vi "OL_WaveSaver_rt.vi"() -> ()   [LabVIEW 2020]
uses:
  <vilib>/FPGAPlugInAG/cRIO-9049/niLvFpga_Open_cRIO-9049.vi
  <vilib>/Utility/error.llb/Error Cluster From Error Code.vi
  <vilib>/rvi/errors/niLvFpgaAdjustHostInterfaceError.vi
  <vilib>/FPGAPlugInAG/cRIO-9049/niLvFpga_Run_cRIO-9049.vi
  <vilib>/FPGAPlugInAG/cRIO-9049/niLvFpga_Close_cRIO-9049.vi
  <vilib>/rvi/interface/nirviOpenFPGA/nirviOpenFPGA.xnode
  FPGA Bitfiles/olwavesaverprj_FPGATarget_OLWaveSaverfpga_hKcI+c2eDyU.lvbitx
  OL_WaveSaver_fpga.vi
  <vilib>/rvi/interface/nirviReadWriteControl/nirviReadWriteControl.xnode
  <vilib>/rvi/interface/nirviMethod/nirviMethod.xnode
  <vilib>/rvi/interface/nirviCloseFPGA/nirviCloseFPGA.xnode
  NiFpgaLv.dll
  <vilib>/FPGAPlugInAG/cRIO-9049/niLvFpga_ReadFifo_cRIO-9049.vi
  <vilib>/rvi/errors/niLvFpgaMergeErrorWithErrorCode.vi
panel:
  in  "Filename":path=path "/home/lvuser/natinst/LABVIEWData/OL_PSD_Map_180.lvm"
  out "0":sgl[](graph)
  out "Sum":sgl[](graph)
  out "Time string":string="11/17/2021 15:18:20.858831"
  out "Filename Out":path=path "/home/lvuser/natinst/LABVIEWData/OL_PSD_Dark_5kHz.lvm"
  in  "decimation":i16=25
  in  "Enable":bool
  out "Saving Data":bool
  out "DeltaX":sgl[](graph)
  out "Elements Remaining":u32
  out "DeltaY":sgl[](graph)
  in  "Number of Elements":u32=400
  in  "stop":bool
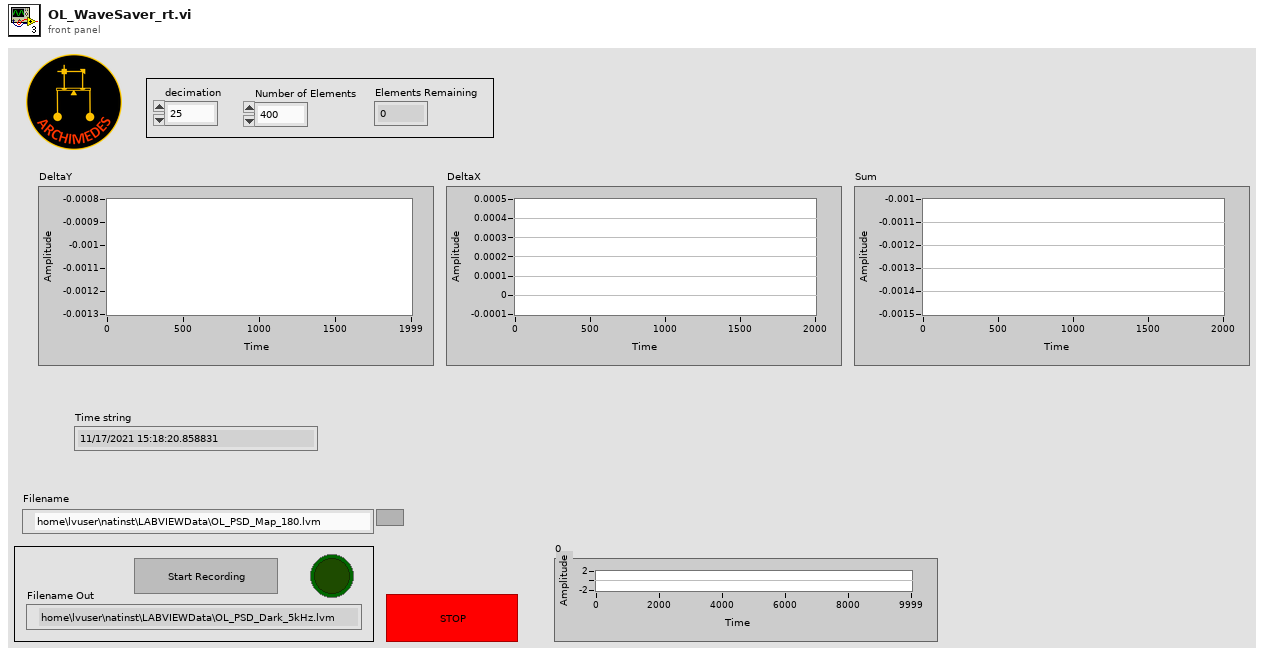
[diagram p1: front panel]
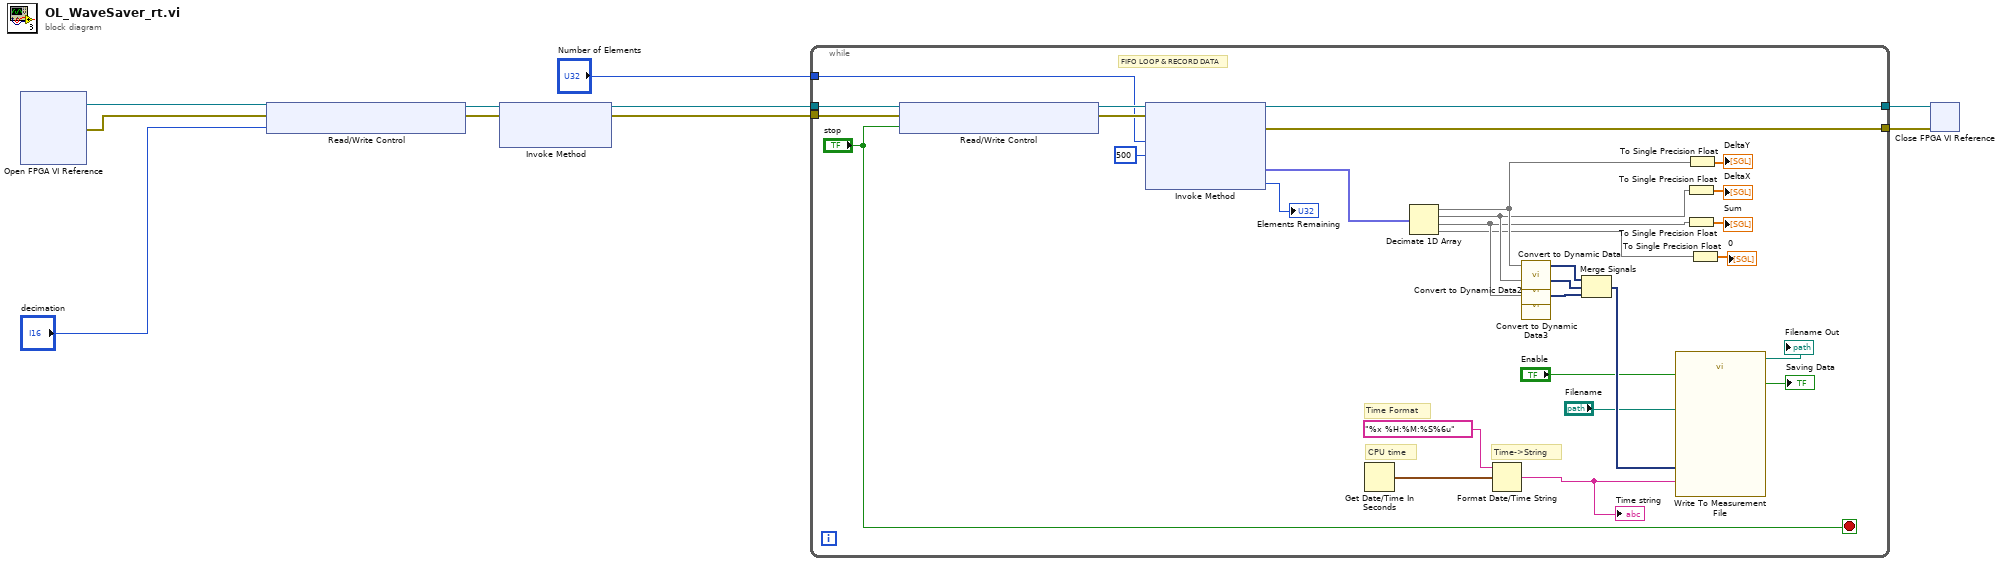
[diagram p0: block diagram]
diagram:
  n1 = xnode "Open FPGA VI Reference"() -> ("FPGA VI Reference Out"=w6:refnum<k20>, "error out"=w5:errorcluster)  [unwired: 2 in]
  n2 = xnode "Read/Write Control"("FPGA VI Reference In"=w6, "error in"=w5, "decimation"="decimation") -> ("FPGA VI Reference Out"=w3:refnum<k20>, "error out"=w2:errorcluster)
  n3 = xnode "Invoke Method"("FPGA VI Reference In"=w3, "error in"=w2) -> ("FPGA VI Reference Out"=w9:refnum<k20>, "error out"=w10:errorcluster)  [unwired: 1 in]
  n4 = while {
    tunnel: w10 -> [w40]
    tunnel: w9 -> [w39]
    tunnel: [w38] -> w8
    tunnel: [w37] -> w4
    tunnel: "Number of Elements" -> [w34]
    stop <- "stop" stop-if-true
    # "FIFO LOOP & RECORD DATA"
    # "Time->String"
    # "CPU time"
    # "Time Format"
    n5 = xnode "Read/Write Control"("FPGA VI Reference In"=w39, "error in"=w40, "stop"="stop") -> ("FPGA VI Reference Out"=w36:refnum<k20>, "error out"=w35:errorcluster)
    n6 = xnode "Invoke Method"("FPGA VI Reference In"=w36, "error in"=w35, "Number of Elements"=w34, "Timeout (ms)"=500) -> ("FPGA VI Reference Out"=w38:refnum<k20>, "error out"=w37:errorcluster, "Data"=w31:fxp<+/-,64,20>[], "Elements Remaining"=→"Elements Remaining":u32)
    n7 = Get Date/Time In Seconds() -> (seconds since 1Jan1904=w25:timestamp)
    n8 = Decimate 1D Array(w31) -> (w22:fxp<+/-,64,20>[], w18:fxp<+/-,64,20>[], w15:fxp<+/-,64,20>[], w13:fxp<+/-,64,20>[])
    n9 = Format Date/Time String(time format string (%c)="%x %H:%M:%S%6u", seconds (now)=w25) -> (date/time string=w19:string)  [unwired: 1 in]
    "Time string" <- w19
    n10 = call "Convert to Dynamic Data"("Array"=w22) -> ("Dynamic Data Type"=w30:dynamicdata)  [unwired: 3 in]
    n11 = call "Convert to Dynamic Data2"("Array"=w18) -> ("Dynamic Data Type"=w29:dynamicdata)  [unwired: 3 in]
    n12 = call "Convert to Dynamic Data3"("Array"=w15) -> ("Dynamic Data Type"=w27:dynamicdata)  [unwired: 3 in]
    n13 = Merge Signals(w30, w29, w27) -> (w28:dynamicdata)
    n14 = call "Write To Measurement File"("Signals"=w28, "Enable"="Enable", "Filename"="Filename", "Comment"=w19) -> ("Filename Out"=→"Filename Out":path, "Saving Data"=→"Saving Data":bool)  [unwired: 13 in, 1 out]
    n15 = To Single Precision Float(number=w18) -> (single precision float=→"DeltaX":sgl[])
    n16 = To Single Precision Float(number=w15) -> (single precision float=→"Sum":sgl[])
    n17 = To Single Precision Float(number=w22) -> (single precision float=→"DeltaY":sgl[])
    n18 = To Single Precision Float(number=w13) -> (single precision float=→"0":sgl[])
  }
  n19 = xnode "Close FPGA VI Reference"("FPGA VI Reference In"=w8, "error in"=w4) -> ()  [unwired: 1 out]
